vi "Get Alias String.vi"(8 "error in (no error)":errorcluster, 11 "Multi Instrument Msg in":refnum<class "Multi Instrument Msg.lvclass">) -> (0 "error out":errorcluster, 2 "Instrument List":string, 3 "Multi Instrument Msg out":refnum<class "Multi Instrument Msg.lvclass">)   [LabVIEW 2020, in "Instrument Handler.lvlib" / "Multi Instrument Msg.lvclass"]
doc: "List all owned alias' in a comma seperated string."
uses:
  Multi Instrument Msg.lvclass
  Multi Instrument Msg.lvclass/Multi Instrument Msg.ctl
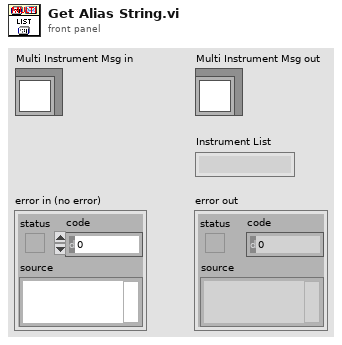
[diagram p1: front panel]
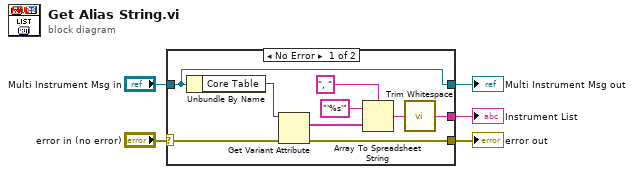
[diagram p0: block diagram]
diagram:
  n1 = case shown="No Error" "error in (no error)" {
    selector: "error in (no error)" -> [w11 w16]
    tunnel: [w10 w16] -> w4
    tunnel: [w14 w15] -> w2
    tunnel: "Multi Instrument Msg in" -> [w14 w15]
    tunnel: [w6 _] -> w1
    frame No Error {
      n2 = Unbundle By Name(w14) -> ("Core Table"=w13:variant)
      n3 = Get Variant Attribute(Variant=w13, error in=w11) -> (names=w12:string[], error out=w10:errorcluster)  [unwired: 2 in, 2 out]
      n4 = Array To Spreadsheet String(delimiter (Tab)=", ", array=w12, 3:"'%s'" ("format string")) -> (spreadsheet string=w7:string)
      n5 = call <vilib>:"Trim Whitespace.vi"("string"=w7) -> ("trimmed string"=w6:string)  [unwired: 1 in]
    }
    frame Error {
    }
  }
  "error out" <- w4
  "Multi Instrument Msg out" <- w2
  "Instrument List" <- w1
